vi "run.vi"(8 "error in (no error)":errorcluster, 11 "ImagingModeMG091111IntrinsicImaging in":refnum<class "ImagingModeMG091111IntrinsicImaging.lvclass">) -> (0 "error out":errorcluster, 3 "ImagingModeMG091111IntrinsicImaging out":refnum<class "ImagingModeMG091111IntrinsicImaging.lvclass">)   [LabVIEW 2010, in "ImagingModeMG091111IntrinsicImaging.lvclass"]
uses:
  ImagingModeMG091111IntrinsicImaging.lvclass
  common/xcontrols/XSettings/XSettings/XSettings.xctl
  common/classes/GenericComponent/GenericComponent/GenericComponent.lvclass
  main/labview_source/controls/undock_button.ctl
  ImagingModeMG091111IntrinsicImaging.lvclass/ImagingModeMG091111IntrinsicImaging.ctl
  ImagingModeDL091001Scaffold/ImagingModeDL091001Scaffold/ImagingModeDL091001Scaffold.lvclass
  ImagingModeDL091001Scaffold/ImagingModeDL091001Scaffold/internal_triggers_enum.ctl
  common/classes/ErrorController/ErrorController/class_data.vi
  GenericImagingMode/GenericImagingMode/GenericImagingMode.lvclass
  common/classes/ErrorController/ErrorController/ErrorController.lvclass
panel:
  out "settings enforced?":bool
  in  "button:undock":T1
  in  "Tab Control":enum32{"User", "About"}(tab)
  in  "frame rate":dbl[unit]=5.0
  in  "image height":i32=200
  in  "image width":i32=200
  in  "offset time":dbl[unit]=0.5
  in  "phase duration":dbl[unit]=5.0
  in  "skip control":bool
  in  "XSettings":refnum<class "GenericComponent.lvclass">(xcontrol)
  out "finished?":bool
  # "ImagingModeMG091111IntrinsicImaging\n\nImplemented by:\nMaurice Göldi and Dominik Langer, University of Zurich, Switzerland"
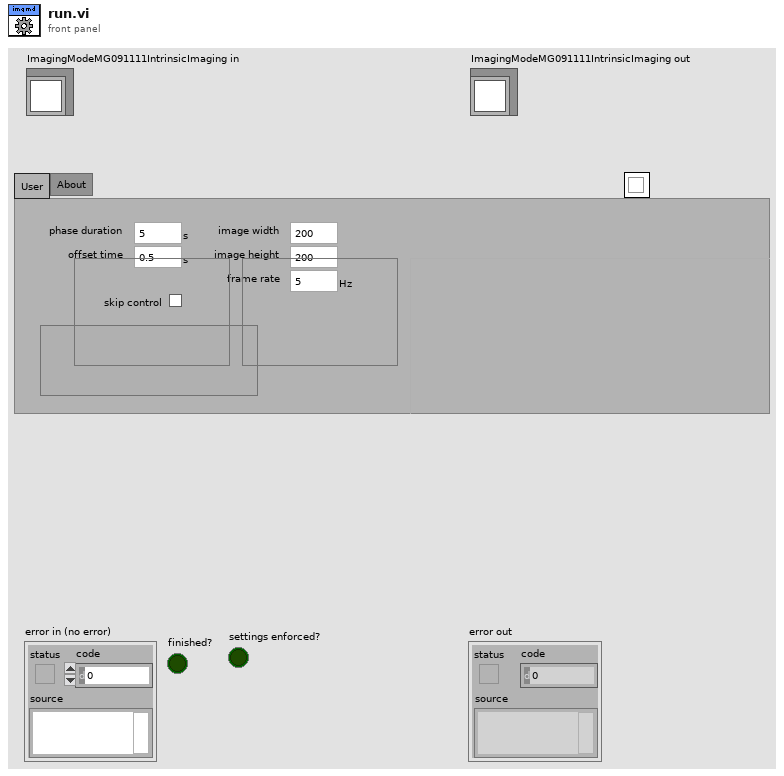
[diagram p1: front panel]
types:
  T1 = typedef "undock_button.ctl" = bool
  T2 = typedef "ImagingModeDL091001Scaffold.lvclass/internal_triggers_enum.ctl" = enum16{"NULL", "initialise", "terminate", "start sweep", "stop sweep", "update", "proceed", "draw overlay", "attach observer", "detach observer", "finish sweep"}
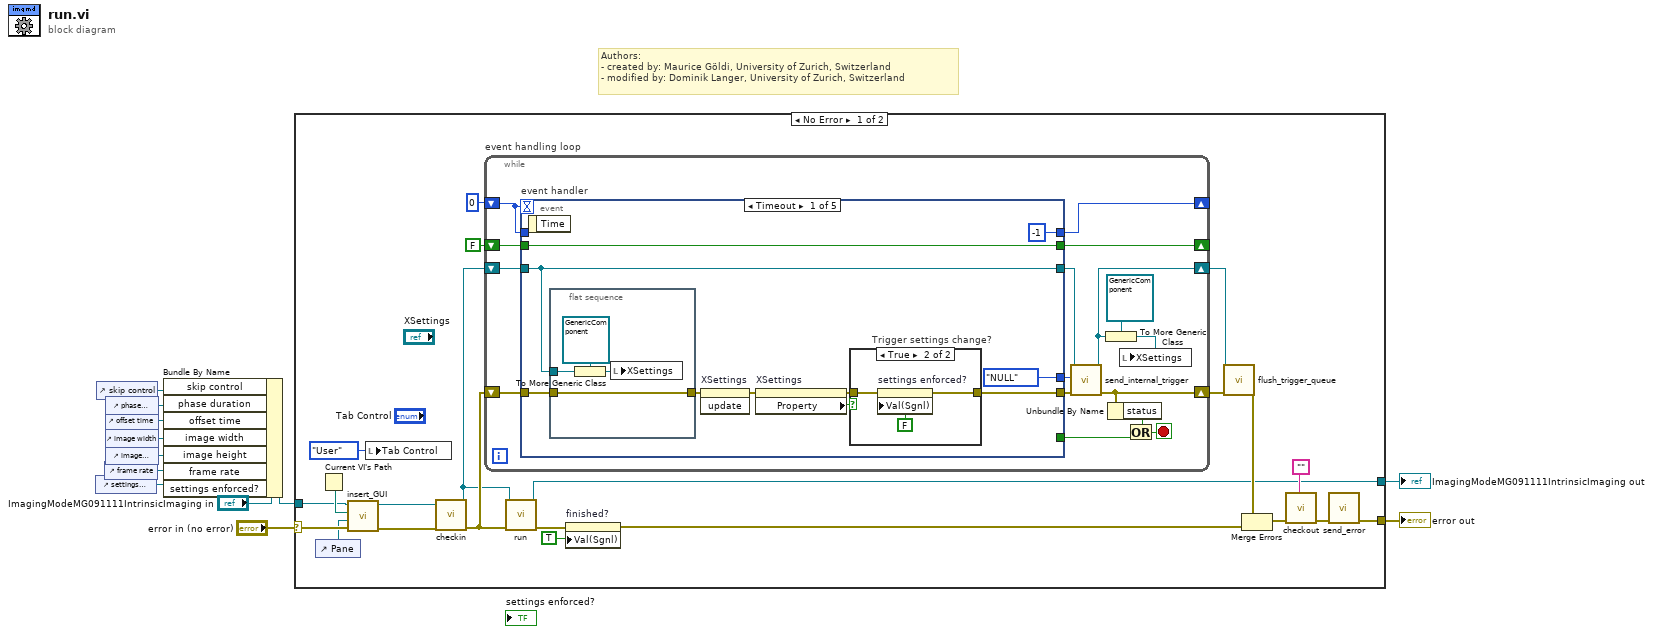
[diagram p0: block diagram]
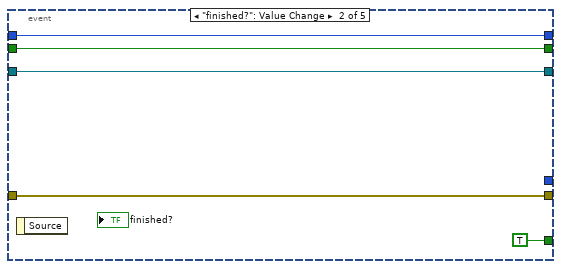
[diagram p3: hidden frame]
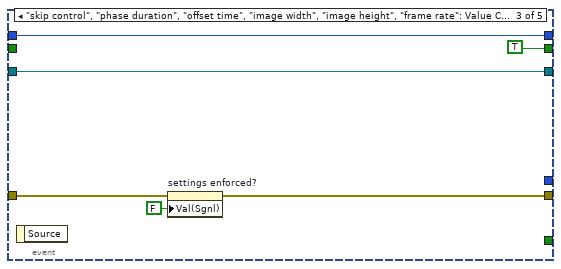
[diagram p4: hidden frame]
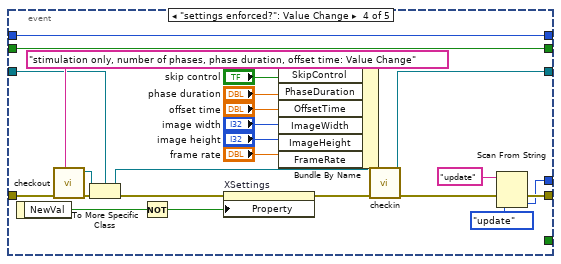
[diagram p5: hidden frame]
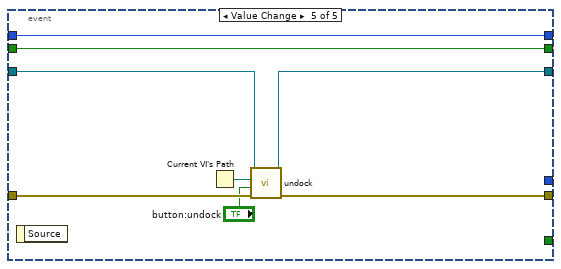
[diagram p6: hidden frame]
diagram:
  # "Authors: \n- created by: Maurice Göldi, University of Zurich, Switzerland\n- modified by: Dominik Langer, University of Zurich, Switzerland"
  n1 = control-ref of="settings enforced?"() -> (w1:refnum<vi>)
  n2 = control-ref of="skip control"() -> (w4:refnum<vi>)
  n3 = control-ref of="frame rate"() -> (w9:refnum<vi>)
  n4 = control-ref of="phase duration"() -> (w5:refnum<vi>)
  n5 = control-ref of="offset time"() -> (w6:refnum<vi>)
  n6 = control-ref of="image width"() -> (w7:refnum<vi>)
  n7 = control-ref of="image height"() -> (w8:refnum<vi>)
  n8 = Bundle By Name(cluster="ImagingModeMG091111IntrinsicImaging in", "skip control"=w4, "phase duration"=w5, "offset time"=w6, "image width"=w7, "image height"=w8, "frame rate"=w9, "settings enforced?"=w1) -> (w2:refnum<class "ImagingModeMG091111IntrinsicImaging.lvclass">)
  n9 = case shown="No Error" "error in (no error)" {
    selector: "error in (no error)" -> [w27 w114]
    tunnel: [w14 w114] -> w12
    tunnel: [w13 w113] -> w11
    tunnel: w2 -> [w25 w113]
    frame No Error {
      n10 = control-ref of="Pane"() -> (w24:refnum<vi>)
      n11 = Current VI's Path() -> (path=w26:path)
      n12 = call-dynamic "insert_GUI.vi"("error in (no error)"=w27, "Pane"=w24, "VI path"=w26, "GenericComponent in"=w25) -> ("error out"=w19:errorcluster, "GenericComponent out"=w18:refnum<class "ImagingModeMG091111IntrinsicImaging.lvclass">)  [unwired: 6 in]
      n13 = local write "Tab Control"(enum32{"User", "About"}."User" ("Tab Control")) -> ()
      n14 = call-dynamic "checkin.vi"("error in (no error)"=w19, "GenericScanMode in"=w18) -> ("error out"=w32:errorcluster, "GenericScanMode out"=w16:refnum<class "ImagingModeMG091111IntrinsicImaging.lvclass">)  [unwired: 8 in]
      n15 = while "event handling loop" {
        shift-right: [w49] -> _
        shift-left: 0 -> [w50]
        shift-right: [w43] -> w21
        shift-left: w32 -> [w48]
        shift-right: [w45] -> _
        shift-left: FALSE -> [w46]
        shift-right: [w35] -> w17
        shift-left: w16 -> [w47]
        stop <- w40 stop-if-true
        n16 = event "event handler" shown="[0] Timeout" {
          selector: _ -> [_ _ _ _ _]
          dyn-events: _ -> [_ _ _ _ _]
          timeout: w50 -> [_ _ _ _ _]
          tunnel: w50 -> [_ w73 w79 w104 w112]
          tunnel: [-1 w73 w79 w104 w112] -> w49
          tunnel: w48 -> [w57 w72 w77 w87 w110]
          tunnel: [w54 w72 w76 w85 w109] -> w44
          tunnel: [_ TRUE _ _ _] -> w42
          tunnel: [internal_triggers_enum."NULL" ("trigger") _ _ w84 _] -> w38
          tunnel: w47 -> [w56 w69 w74 w86 w108]
          tunnel: w46 -> [w59 w70 _ w103 w111]
          tunnel: [w59 w70 TRUE w103 w111] -> w45
          tunnel: [w56 w69 w74 w82 w107] -> w39
          event Timeout {
            n17 = event-data() -> ()  [unwired: 1 in, 1 out]
            n18 = flat-sequence {
              tunnel: w57 -> [w65]
              tunnel: w56 -> [w67]
              tunnel: [w65] -> w53
              frame #0 {
                n19 = To More Generic Class(target class=refnum<class "GenericComponent.lvclass"> refnum ("GenericComponent.lvclass"), reference=w67) -> (generic class reference=w68:refnum<class "GenericComponent.lvclass">)
                n20 = local write "XSettings"(w68) -> ()
              }
            }
            n21 = invoke on="XSettings" class="XSettings (strict)" method="update"(error in=w53) -> (error out=w52:errorcluster)  [unwired: 2 in, 2 out]
            n22 = property on="XSettings" class="XSettings (strict)"(error in=w52) -> (error out=w55:errorcluster, "Property"=w51:bool)  [unwired: 1 in, 1 out]
            n23 = case "Trigger settings change?" shown="True" w51 {
              tunnel: w55 -> [w61 w64]
              tunnel: [w61 w63] -> w54
              frame False {
              }
              frame True {
                n24 = property on="settings enforced?" class="Bool (strict)"(error in=w64, "Val(Sgnl)"=FALSE) -> (error out=w63:errorcluster)  [unwired: 1 in, 1 out]
              }
            }
          }
          event "finished?": Value Change {
            n25 = event-data() -> ()  [unwired: 1 in, 1 out]
          }
          event "skip control", "phase duration", "offset time", "image width", "image height", "frame rate": Value Change {
            n26 = event-data() -> ()  [unwired: 1 in, 1 out]
            n27 = property on="settings enforced?" class="Bool (strict)"(error in=w77, "Val(Sgnl)"=FALSE ("settings enforced?")) -> (error out=w76:errorcluster)  [unwired: 1 in, 1 out]
          }
          event "settings enforced?": Value Change {
            n28 = event-data() -> ("NewVal"=w81:bool)  [unwired: 1 in]
            n29 = call "checkout.vi"("locked by?"="stimulation only, number of phases, phase duration, offset time: Value Change", "error in (no error)"=w87) -> ("error out"=w99:errorcluster, "GenericScanMode out"=w98:refnum<class "GenericImagingMode.lvclass">)  [unwired: 8 in]
            n30 = To More Specific Class(target class=w86, reference=w98, error in=w99) -> (specific class reference=w97:refnum<class "ImagingModeMG091111IntrinsicImaging.lvclass">, error out=w89:errorcluster)
            n31 = Not(x=w81) -> (.not. x?=w80:bool)
            n32 = property on="XSettings" class="XSettings (strict)"(error in=w89, "Property"=w80) -> (error out=w88:errorcluster)  [unwired: 1 in, 1 out]
            n33 = Bundle By Name(cluster=w97, "SkipControl"="skip control", "PhaseDuration"="phase duration", "OffsetTime"="offset time", "ImageWidth"="image width", "ImageHeight"="image height", "FrameRate"="frame rate") -> (w96:refnum<class "ImagingModeMG091111IntrinsicImaging.lvclass">)
            n34 = call-dynamic "checkin.vi"("error in (no error)"=w88, "GenericScanMode in"=w96) -> ("error out"=w91:errorcluster, "GenericScanMode out"=w82:refnum<class "ImagingModeMG091111IntrinsicImaging.lvclass">)  [unwired: 8 in]
            n35 = Scan From String(input string="update", error in=w91, default 1=internal_triggers_enum."update" ("trigger")) -> (error out=w85:errorcluster, output 1=w84:T2)  [unwired: 2 in, 2 out]
          }
          event Value Change {
            n36 = event-data() -> ()  [unwired: 1 in, 1 out]
            n37 = Current VI's Path() -> (path=w105:path)
            n38 = call-dynamic "undock.vi"("error in (no error)"=w110, "undock?"="button:undock", "VI path"=w105, "GenericComponent in"=w108) -> ("error out"=w109:errorcluster, "GenericComponent out"=w107:refnum<class "ImagingModeMG091111IntrinsicImaging.lvclass">)  [unwired: 6 in]
          }
        }
        n39 = call-dynamic "send_internal_trigger.vi"("error in"=w44, "trigger"=w38, "ScanModeDL091001Scaffold in"=w39) -> ("error out"=w43:errorcluster, "ScanModeDL091001Scaffold out"=w35:refnum<class "ImagingModeMG091111IntrinsicImaging.lvclass">)  [unwired: 7 in]
        n40 = To More Generic Class(target class=refnum<class "GenericComponent.lvclass"> refnum ("GenericComponent.lvclass"), reference=w35) -> (generic class reference=w37:refnum<class "GenericComponent.lvclass">)
        n41 = Unbundle By Name(w43) -> ("status"=w41:bool)
        n42 = local write "XSettings"(w37) -> ()
        n43 = Or(x=w41, y=w42) -> (x .or. y?=w40:bool)
      }
      n44 = call-parent "run.vi"("error in (no error)"=w32, "ScanModeDL091001Scaffold in"=w16) -> ("error out"=w31:errorcluster, "ScanModeDL091001Scaffold out"=w13:refnum<class "ImagingModeMG091111IntrinsicImaging.lvclass">)  [unwired: 8 in]
      n45 = property on="finished?" class="Bool (strict)"(error in=w31, "Val(Sgnl)"=TRUE) -> (error out=w30:errorcluster)  [unwired: 1 in, 1 out]
      n46 = call-dynamic "flush_trigger_queue.vi"("error in (no error)"=w21, "GenericToplevelComponent in"=w17) -> ("error out"=w20:errorcluster)  [unwired: 8 in, 1 out]
      n47 = Merge Errors(w20, w30) -> (w29:errorcluster)
      n48 = call "checkout.vi"("locked by?"="", "error in (no error)"=w29) -> ("error out"=w15:errorcluster)  [unwired: 8 in, 1 out]
      n49 = call "send_error.vi"("error in (no error)"=w15) -> ("error out"=w14:errorcluster)  [unwired: 10 in]
    }
    frame Error {
    }
  }
  "error out" <- w12
  "ImagingModeMG091111IntrinsicImaging out" <- w11
